vi "FPGA Top Level.vi"() -> ()   [LabVIEW 2017]
uses:
  <vilib>/Platform/TimedLoop/XDataNode/timing_clust.ctl
  <vilib>/Platform/TimedLoop/XDataNode/nitl_modes.ctl
  <vilib>/Platform/TimedLoop/XDataNode/wakeup.ctl
  <vilib>/rvi/Emulation/niFpgaGetClockAttributes.vi
  <vilib>/rvi/Emulation/niFpgaSctlEmulationGetInTimedLoop.vi
  <vilib>/rvi/Emulation/niFpgaEmulationReportErrorSimple.vi
  <vilib>/rvi/Emulation/niFpgaProcessEmulError.vi
  <vilib>/rvi/eio/common/nirviEmuTemplateMethod_errors.vi
  <vilib>/rvi/Emulation/niFpgaCriticalErrorInLSC.vi
  <vilib>/eio/EIONode/EIONode.xnode
  <vilib>/Platform/TimedLoop/XDataNode/XDataNode.xnode
  <vilib>/Platform/TimedLoop/XDataNode/XDNodeRunTimeDep.lvlib
panel:
  out "Link 1 PWM Duty (Counts)":i32
  out "Link 2 PWM Duty (Counts)":i32
  in  "Enable motor 2":bool
  in  "Enable motor 1":bool
  in  "Link 1 Direction":bool
  in  "Link 2 Direction":bool
  in  "Link 1 Demand":fxp<+/-,32,8>
  in  "Link 2 Demand":fxp<+/-,32,8>
  in  "PWM Period Loops":i32=200
  out "PWM Period (ticks)":u32
  in  "PWM Gen Period (ms)":u16=10
  # "Motor Data"
  # "PWM Data"
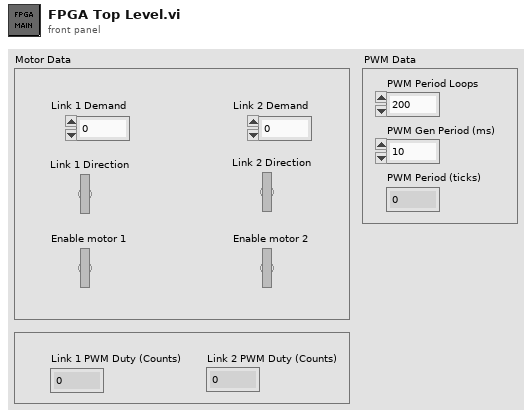
[diagram p1: front panel]
types:
  T1 = typedef "XDNodeRunTimeDep.lvlib/timing_clust.ctl" = cluster{"Expected End [f-1]":u64, "Actual End [f-1]":u64, "Finished Late? [f-1]":bool, "Expected End [i-1]":u64, "Actual End [i-1]":u64, "Finished Late? [i-1]":bool, "Expected Start [i]":u64, "Actual Start [i]":u64, "Expected Start [f]":u64, "Actual Start [f]":u64, "Source Name":string, "Structure Name":string, "Period":i64, "Deadline":i64, "Offset":i64, "Start":i64, "Priority":i32, "Timeout":i32, "Mode":T2, "Wakeup Reason":T3, "Error":errorcluster, "Source Type":string, "Secondary Source Type":string, "Global End Time":u64, "Global Start Time":u64, "Frame Duration":u64, "Iteration Duration":u64, "Assigned CPU":i32, "I/O Scan Engine Mode":u32}
  T2 = typedef "XDNodeRunTimeDep.lvlib/nitl_modes.ctl" = enum32{"No Change", "Process missed periods, maintain original phase", "Discard missed periods, maintain original phase", "Process missed periods, ignore original phase", "Discard missed periods, ignore original phase"}
  T3 = typedef "XDNodeRunTimeDep.lvlib/wakeup.ctl" = enum32{"Normal", "Aborted", "Asynchronous wakeup", "Timing source error", "Timed loop error", "Timeout"}
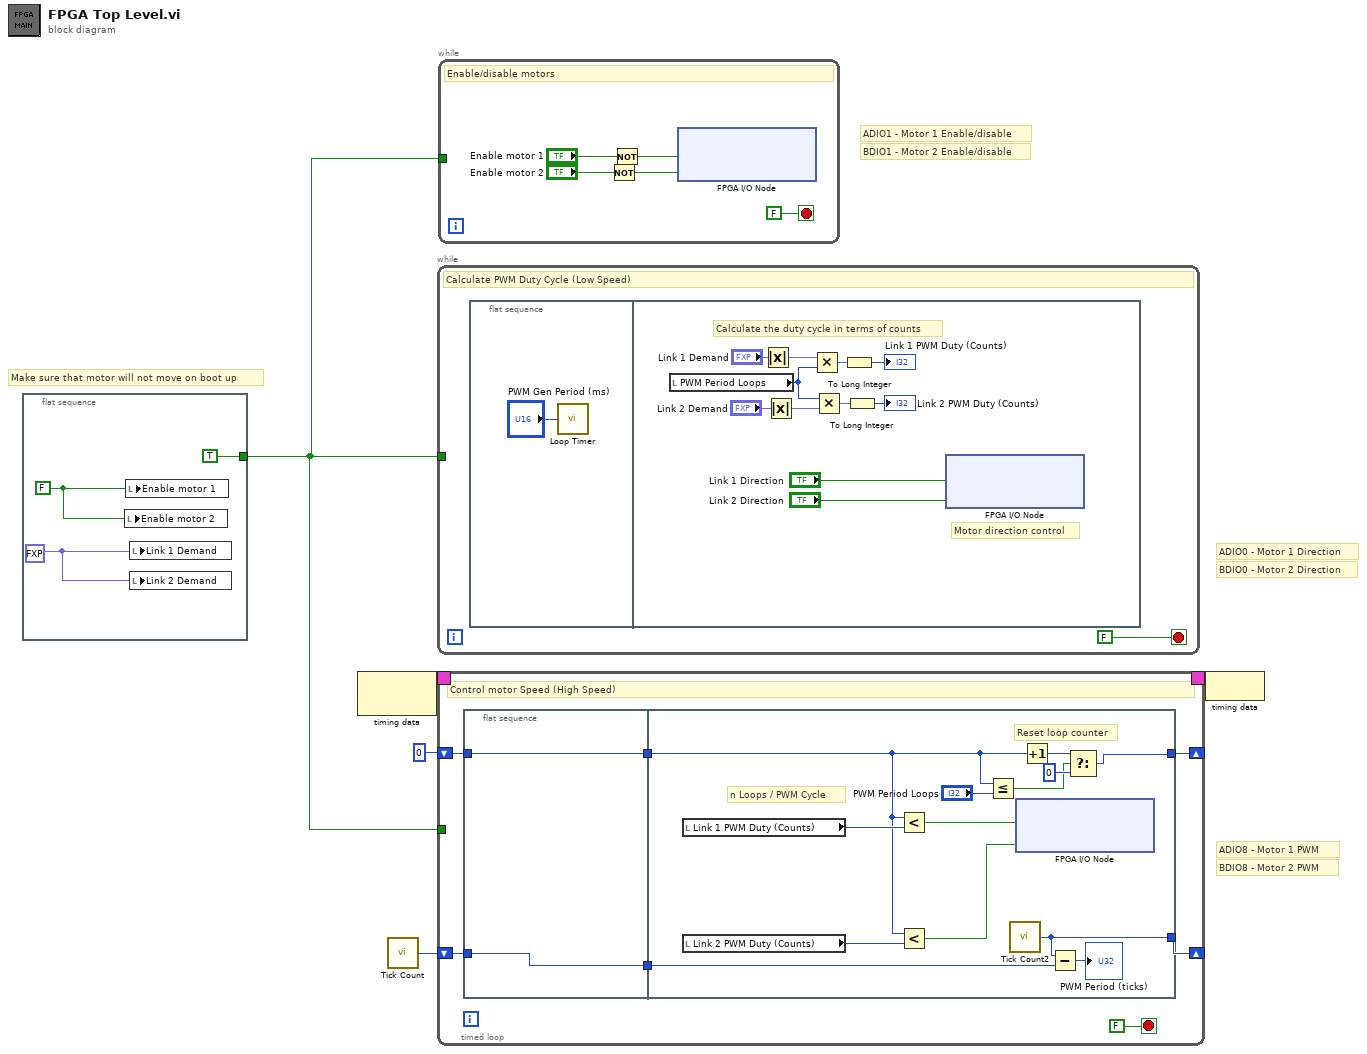
[diagram p0: block diagram]
diagram:
  # "BDIO1 - Motor 2 Enable/disable"
  # "ADIO1 - Motor 1 Enable/disable"
  # "BDIO0 - Motor 2 Direction"
  # "ADIO0 - Motor 1 Direction"
  # "BDIO8 - Motor 2 PWM"
  # "ADIO8 - Motor 1 PWM"
  # "Make sure that motor will not move on boot up"
  n1 = flat-sequence {
    tunnel: [TRUE] -> w1
    frame #0 {
      w6 = FALSE
      w8 = fxp<+/-,32,0> 0.0 ("Link_1 Duty")
      n2 = local write "Enable motor 2"(w6) -> ()
      n3 = local write "Enable motor 1"(w6) -> ()
      n4 = local write "Link 1 Demand"(w8) -> ()
      n5 = local write "Link 2 Demand"(w8) -> ()
    }
  }
  n6 = node-c288() -> (w5:T1)  [unwired: 1 in]
  n7 = call "Tick Count"() -> ("Tick Count(Ticks)"=w3:u32)
  n8 = while {
    tunnel: w1 -> [_]
    stop <- FALSE stop-if-true
    # "Calculate PWM Duty Cycle (Low Speed)"
    n9 = flat-sequence {
      frame #0 {
        n10 = call "Loop Timer"("Count(mSec)"="PWM Gen Period (ms)") -> ()  [unwired: 1 out]
      }
      frame #1 {
        # "Motor direction control"
        # "Calculate the duty cycle in terms of counts"
        n11 = local read "PWM Period Loops"() -> (w15:i32)
        n12 = Absolute Value(x="Link 1 Demand") -> (abs(x)=w19:fxp<+,32,8>)
        n13 = Absolute Value(x="Link 2 Demand") -> (abs(x)=w16:fxp<+,32,8>)
        n14 = Multiply(x=w19, y=w15) -> (x*y=w20:fxp<+/-,63,39>)
        n15 = Multiply(x=w15, y=w16) -> (x*y=w18:fxp<+/-,63,39>)
        n16 = To Long Integer(number=w20) -> (32bit integer=→"Link 1 PWM Duty (Counts)":i32)
        n17 = To Long Integer(number=w18) -> (32bit integer=→"Link 2 PWM Duty (Counts)":i32)
        n18 = xnode "FPGA I/O Node"("ConnectorA/DIO0"="Link 1 Direction", "ConnectorB/DIO0"="Link 2 Direction") -> ()  [unwired: 2 in, 2 out]
      }
    }
  }
  n19 = timed-loop {
    shift-right: [w27] -> _
    shift-left: w3 -> [w26]
    timing: w5 -> [_]
    timing-out: [_] -> w4
    shift-right: [w24] -> _
    shift-left: i16 0 -> [w23]
    tunnel: w1 -> [_]
    stop <- FALSE stop-if-true
    # "Control motor Speed (High Speed)"
    n20 = flat-sequence {
      tunnel: w26 -> [w30]
      tunnel: [w30] -> w25
      tunnel: w23 -> [w29]
      tunnel: [w29] -> w22
      tunnel: [w39] -> w27
      tunnel: w25 -> [w38]
      tunnel: [w35] -> w24
      tunnel: w22 -> [w32]
      frame #0 {
      }
      frame #1 {
        # "Reset loop counter"
        # "n Loops / PWM Cycle"
        n21 = local read "Link 1 PWM Duty (Counts)"() -> (w41:i32)
        n22 = local read "Link 2 PWM Duty (Counts)"() -> (w40:i32)
        n23 = Less?(x=w32, y=w41) -> (x < y?=w43:bool)
        n24 = Less?(x=w32, y=w40) -> (x < y?=w42:bool)
        n25 = Less Or Equal?(x=w32, y="PWM Period Loops") -> (x <= y?=w31:bool)
        n26 = call "Tick Count2"() -> ("Tick Count(Ticks)"=w39:u32)
        n27 = xnode "FPGA I/O Node"("ConnectorA/DIO8"=w43, "ConnectorB/DIO8"=w42) -> ()  [unwired: 2 in, 2 out]
        n28 = Increment(x=w32) -> (x+1=w36:i16)
        n29 = Subtract(x=w39, y=w38) -> (x-y=→"PWM Period (ticks)":u32)
        n30 = Select(t=w36, s=w31, f=i16 0) -> (s? t:f=w35:i16)
      }
    }
  }
  n31 = while {
    tunnel: w1 -> [_]
    stop <- FALSE stop-if-true
    # "Enable/disable motors"
    n32 = Not(x="Enable motor 2") -> (.not. x?=w46:bool)
    n33 = Not(x="Enable motor 1") -> (.not. x?=w47:bool)
    n34 = xnode "FPGA I/O Node"("ConnectorA/DIO1"=w47, "ConnectorB/DIO1"=w46) -> ()  [unwired: 2 in, 2 out]
  }
  n35 = node-c288(w4) -> ()
